vi "Pre-Uninstall Custom Action - Generator.vi"() -> (0 "error out":errorcluster)   [LabVIEW 2021]
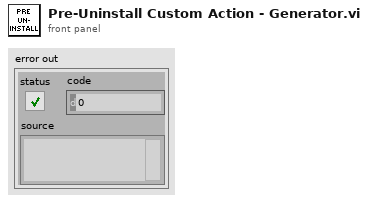
[diagram p1: front panel]
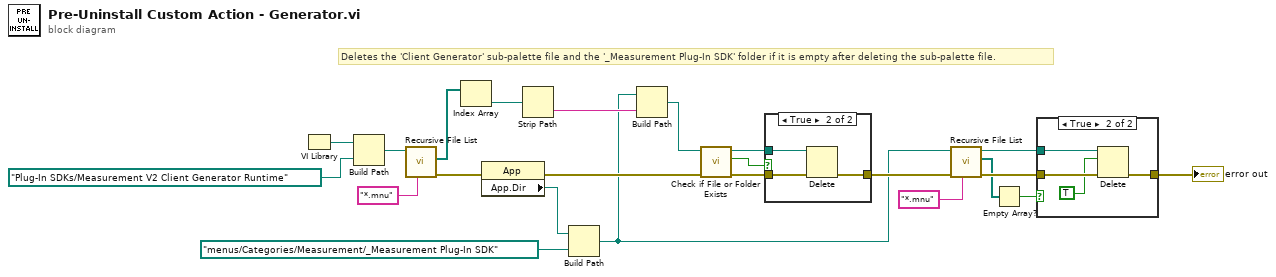
[diagram p0: block diagram]
diagram:
  # "Deletes the 'Client Generator' sub-palette file and the '_Measurement Plug-In SDK' folder if it is empty after deleting the sub-palette file."
  n1 = VI Library() -> (path=w8:path)
  n2 = Build Path(base path=w8, name or relative path=path "Plug-In SDKs/Measurement V2 Client Generator Runtime") -> (appended path=w23:path)
  n3 = call <vilib>:"Recursive File List.vi"("pattern"="*.mnu", "Folder Path"=w23) -> ("error out"=w17:errorcluster, "All Files in Dir"=w21:path[])  [unwired: 5 in, 3 out]
  n4 = Index Array(array=w21) -> (element=w16:path)  [unwired: 1 in]
  n5 = property class="App"(error in=w17) -> (error out=w20:errorcluster, "App.Dir"=w19:path)  [unwired: 1 in, 1 out]
  n6 = Strip Path(path=w16) -> (name=w15:string)  [unwired: 1 out]
  n7 = Build Path(base path=w19, name or relative path=path "menus/Categories/Measurement/_Measurement Plug-In SDK") -> (appended path=w6:path)
  n8 = Build Path(base path=w6, name or relative path=w15) -> (appended path=w14:path)
  n9 = call <vilib>:"Check if File or Folder Exists.vi"("error in (no error)"=w20, "path"=w14) -> ("error out"=w13:errorcluster, "file or folder exists?"=w12:bool, "dup path"=w11:path)  [unwired: 7 in]
  n10 = case shown="True" w12 {
    tunnel: [w24 w27] -> w10
    tunnel: w13 -> [w24 w26]
    tunnel: w11 -> [_ w25]
    frame False {
    }
    frame True {
      n11 = Delete(path (use dialog)=w25, error in=w26) -> (error out=w27:errorcluster)  [unwired: 3 in, 2 out]
    }
  }
  n12 = call <vilib>:"Recursive File List.vi"("pattern"="*.mnu", "error in (no error)"=w10, "Folder Path"=w6) -> ("error out"=w7:errorcluster, "All Files in Dir"=w4:path[], "dup Folder Path"=w2:path)  [unwired: 4 in, 2 out]
  n13 = Empty Array?(array=w4) -> (empty?=w1:bool)
  n14 = case shown="True" w1 {
    tunnel: w7 -> [w28 w32]
    tunnel: [w28 w31] -> w3
    tunnel: w2 -> [_ w30]
    frame False {
    }
    frame True {
      n15 = Delete(path (use dialog)=w30, entire hierarchy (F)=TRUE, error in=w32) -> (error out=w31:errorcluster)  [unwired: 2 in, 2 out]
    }
  }
  "error out" <- w3
